vi "未命名 1.vi"() -> ()   [LabVIEW 2018]
panel:
  out "OutData":string[](array[string])
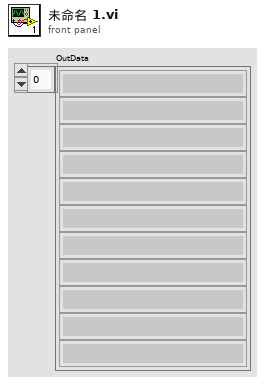
[diagram p1: front panel]
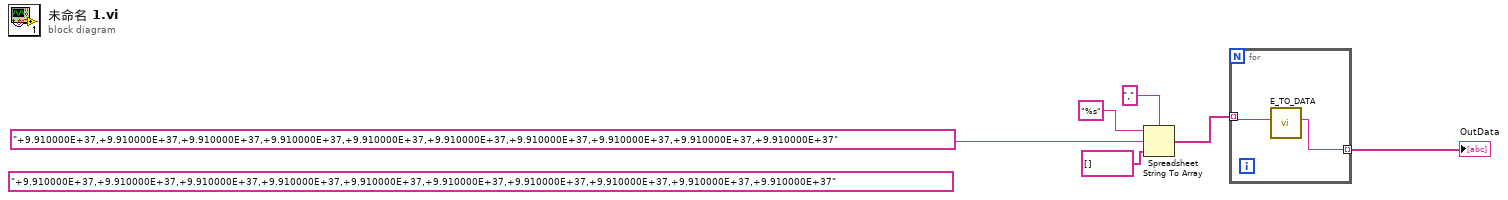
[diagram p0: block diagram]
diagram:
  (unwired) "+9.910000E+37,+9.910000E+37,+9.910000E+37,+9.910000E+37,+9.910000E+37,+9.910000E+37,+9.910000E+37,+9.910000E+37,+9.910000E+37,+9.910000E+37"
  n1 = Spreadsheet String To Array(delimiter (Tab)="," ("分隔符(Tab)"), format string="%s" ("电子表格字符串"), spreadsheet string="+9.910000E+37,+9.910000E+37,+9.910000E+37,+9.910000E+37,+9.910000E+37,+9.910000E+37,+9.910000E+37,+9.910000E+37,+9.910000E+37,+9.910000E+37", array type (2D Dbl)=string[] []) -> (array=w5:string[])
  n2 = for {
    tunnel: w5 -> [w8] mode=indexing
    tunnel: [w7] -> w6 mode=indexing
    n3 = call "E_TO_DATA.vi"("INPUT"=w8) -> ("F-格式字符串"=w7:string)  [unwired: 10 in]
  }
  "OutData" <- w6
